vi "aft_xmpl_Decision.vi"(11 "y(n)":cdb) -> (2 "successful?":bool, 3 "d(n)":cdb)   [LabVIEW 2023]
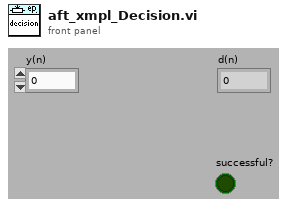
[diagram p1: front panel]
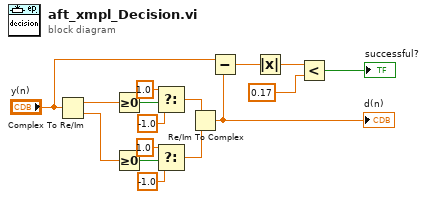
[diagram p0: block diagram]
diagram:
  n1 = Complex To Re/Im(x + iy="y(n)") -> (x=w16:dbl, y=w9:dbl)
  n2 = Greater Or Equal To 0?(x=w16) -> (x >= 0?=w15:bool)
  n3 = Greater Or Equal To 0?(x=w9) -> (x >= 0?=w12:bool)
  n4 = Select(t=1.0, s=w15, f=-1.0) -> (s? t:f=w8:dbl)
  n5 = Select(t=1.0, s=w12, f=-1.0) -> (s? t:f=w7:dbl)
  n6 = Re/Im To Complex(1:w7, 2:w8) -> (0:w5:cdb)
  "d(n)" <- w5
  n7 = Subtract(x="y(n)", y=w5) -> (x-y=w4:cdb)
  n8 = Absolute Value(x=w4) -> (abs(x)=w3:dbl)
  n9 = Less?(x=w3, y=0.17) -> (x < y?=→"successful?":bool)
